vi "Revision Query.vi"(8 "error in (no error)":errorcluster, 9 "Device and Axis":string, 11 "VISA resource name":refnum<visa-resource-name>) -> (0 "error out":errorcluster, 1 "Instrument Firmware Revision":string, 2 "Instrument Driver Revision":string, 3 "VISA resource name out":refnum<visa-resource-name>)   [LabVIEW 2012, in "Zaber A Series.lvlib"]
doc: "Queries the firmware version of the controller as well as the revision of the instrument driver. \n\nThis VI requires that the Initialize VI has been called with the same serial port. \n\nRefer to the Readme file for detailed driver information including modification history."
uses:
  <instrlib>/Zaber A Series/Zaber A Series.lvlib
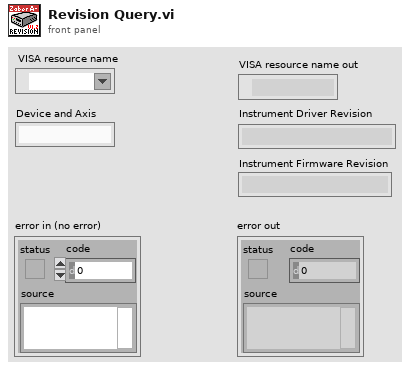
[diagram p1: front panel]
types:
  T1 = cluster{"Major":u16, "Minor":u16, "Fix":u16, "Build":u16}
  T2 = cluster{"Device":string, "Axis":string, "Reply Flag":string, "Status":string, "Warning Flags":string, "Data":string}[]
  T3 = cluster{"Device":string, "Axis":string, "Reply Flag":string, "Status":string, "Warning Flags":string, "Data":string}
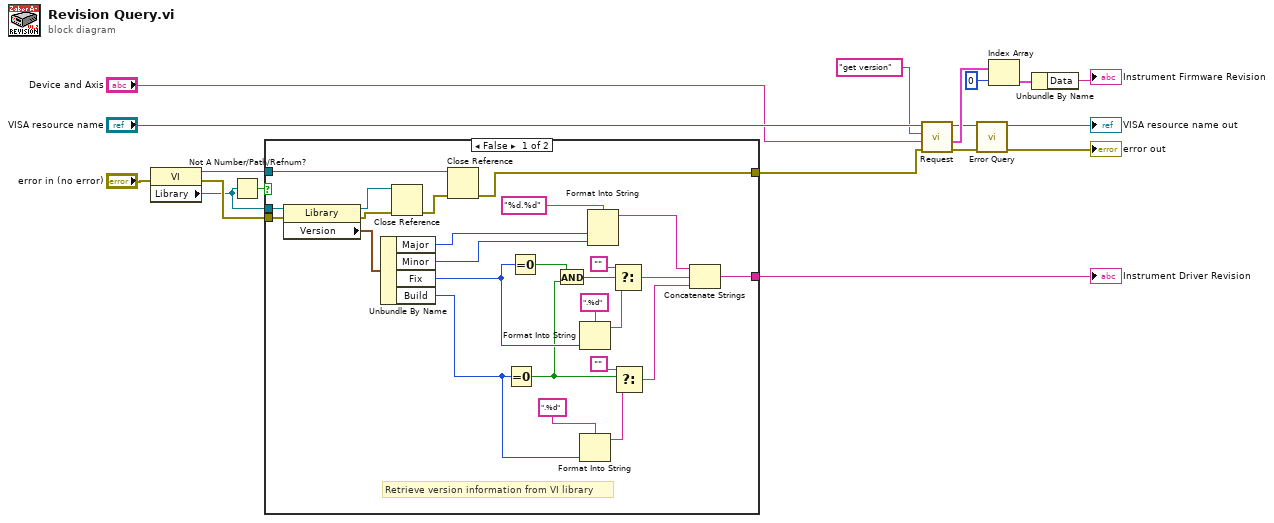
[diagram p0: block diagram]
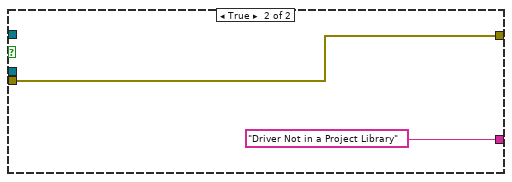
[diagram p2: hidden frame]
diagram:
  n1 = property class="VI"(error in="error in (no error)") -> (reference out=w4:refnum<vi>, error out=w3:errorcluster, "Library"=w2:refnum<vi>)  [unwired: 1 in]
  n2 = Not A Number/Path/Refnum?(number/path/refnum=w2) -> (NaN/Path/Refnum?=w1:bool)
  n3 = case shown="False" w1 {
    tunnel: w4 -> [w41 _]
    tunnel: w3 -> [w26 w46]
    tunnel: [w21 w46] -> w15
    tunnel: [w20 "Driver Not in a Project Library"] -> w16
    tunnel: w2 -> [w19 _]
    frame False {
      # "Retrieve version information from VI library"
      n4 = property class="Library"(reference=w19, error in=w26) -> (reference out=w43:refnum<vi>, error out=w44:errorcluster, "Version"=w40:T1)
      n5 = Unbundle By Name(w40) -> ("Major"=w29:u16, "Minor"=w28:u16, "Fix"=w25:u16, "Build"=w27:u16)
      n6 = Close Reference(reference=w43, error in (no error)=w44) -> (error out=w42:errorcluster)
      n7 = Close Reference(reference=w41, error in (no error)=w42) -> (error out=w21:errorcluster)
      n8 = Equal To 0?(x=w27) -> (x = 0?=w23:bool)
      n9 = Equal To 0?(x=w25) -> (x = 0?=w24:bool)
      n10 = And(x=w24, y=w23) -> (x .and. y?=w22:bool)
      n11 = Format Into String(format string=".%d", w25) -> (resulting string=w37:string)  [unwired: 2 in, 1 out]
      n12 = Format Into String(format string=".%d", w27) -> (resulting string=w33:string)  [unwired: 2 in, 1 out]
      n13 = Format Into String(format string="%d.%d", w29, w28) -> (resulting string=w35:string)  [unwired: 2 in, 1 out]
      n14 = Select(t="", s=w22, f=w37) -> (s? t:f=w34:string)
      n15 = Select(t="", s=w23, f=w33) -> (s? t:f=w30:string)
      n16 = Concatenate Strings(w35, w34, w30) -> (w20:string)
    }
    frame True {
    }
  }
  "Instrument Driver Revision" <- w16
  n17 = call <instrlib>:"Request.vi"("error in (no error)"=w15, "Device and Axis"="Device and Axis", "Command String"="get version", "VISA resource name"="VISA resource name") -> ("error out"=w14:errorcluster, "Response Bundle Array"=w11:T2, "VISA resource name out"=w7:refnum<visa-resource-name>)  [unwired: 3 in, 2 out]
  n18 = call <instrlib>:"Error Query.vi"("error in (no error)"=w14, "VISA resource name"=w7) -> ("error out"=→"error out":errorcluster, "VISA resource name out"=→"VISA resource name out":refnum<visa-resource-name>)  [unwired: 6 in, 2 out]
  n19 = Index Array(array=w11, index=0) -> (element=w9:T3)
  n20 = Unbundle By Name(w9) -> ("Data"=→"Instrument Firmware Revision":string)
